vi "MainRIOEnrique.vi"() -> ()   [LabVIEW 2019]
uses:
  RIOData--cluster.ctl
  Acelerometer data--cluster.ctl
  <vilib>/PantherLAB/Firebase API/PantherLAB_lib_Filtering Parameters--cluster.ctl
  a087fea8-a487-4c1c-8a8b-15f205e78756.vi
  c90b4970-0cb1-4ed8-a3e8-abf7f56642d0.vi
  079ee137-338a-4224-8d27-3950f07d8dd5.vi
  <vilib>/JDP Science/JSONtext/JSON text to Variant.vi
  <vilib>/JDP Science/JSONtext/LVClass Serializer/JSONtext LVClass Serializer.lvclass
  <vilib>/PantherLAB/Firebase API/PantherLAB_lib_firebase.lvclass
  Shared.lvlib
  <vilib>/JDP Science/JSONtext/JSONtext.lvlib
panel:
  in  "Get All":bool
  in  "Get5":bool
  out "JSON String":string
  in  "Get Newest":bool
  in  "Delete":bool
  in  "Password":string="123456"
  in  "Email":string="enrique.noe@gmail.com"
  in  "Log In":bool
  in  "Sign In":bool
  out "Newest":T1
  out "Data out":T1[](array[typedef])
  out "My RIO Acelerometer":T2(graph)
  # "To add an authenticated user\nto your Real Time Database"
  # "If you are already authenticated\nand you want to start using\nyour Database"
  # "Warning:\nThis button will delete all the data\nunder Post EndPoint"
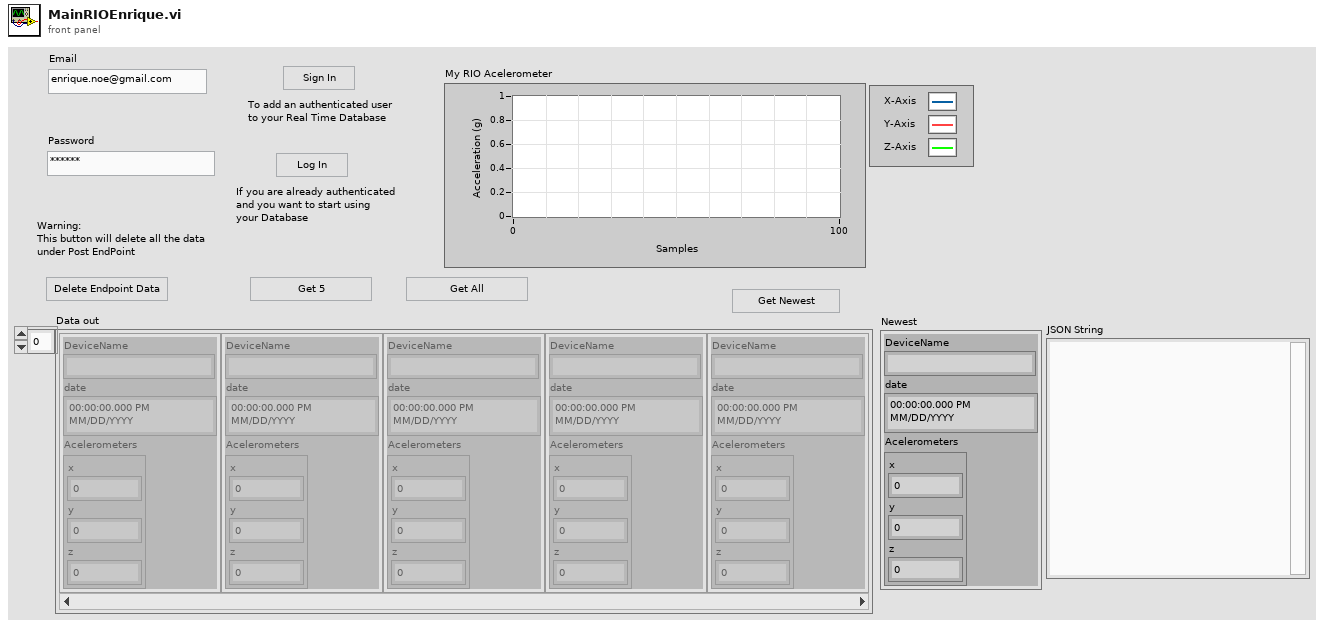
[diagram p1: front panel]
types:
  T1 = typedef "Shared.lvlib/RIOData--cluster.ctl" = cluster{"DeviceName":string, "date":timestamp, "Acelerometers":cluster{"x":dbl, "y":dbl, "z":dbl}}
  T2 = typedef "Shared.lvlib/Acelerometer data--cluster.ctl" = cluster{"X-Axis":dbl, "Y-Axis":dbl, "Z-Axis":dbl}
  T3 = cluster{"Read Access":enum8{"Allowed", "Required", "None"}, "Write Access":enum8{"Allowed", "Required", "None"}}
  T4 = typedef "PantherLAB_lib_firebase.lvclass/PantherLAB_lib_Filtering Parameters--cluster.ctl" = cluster{"Filtering Param":string, "Argument":string}
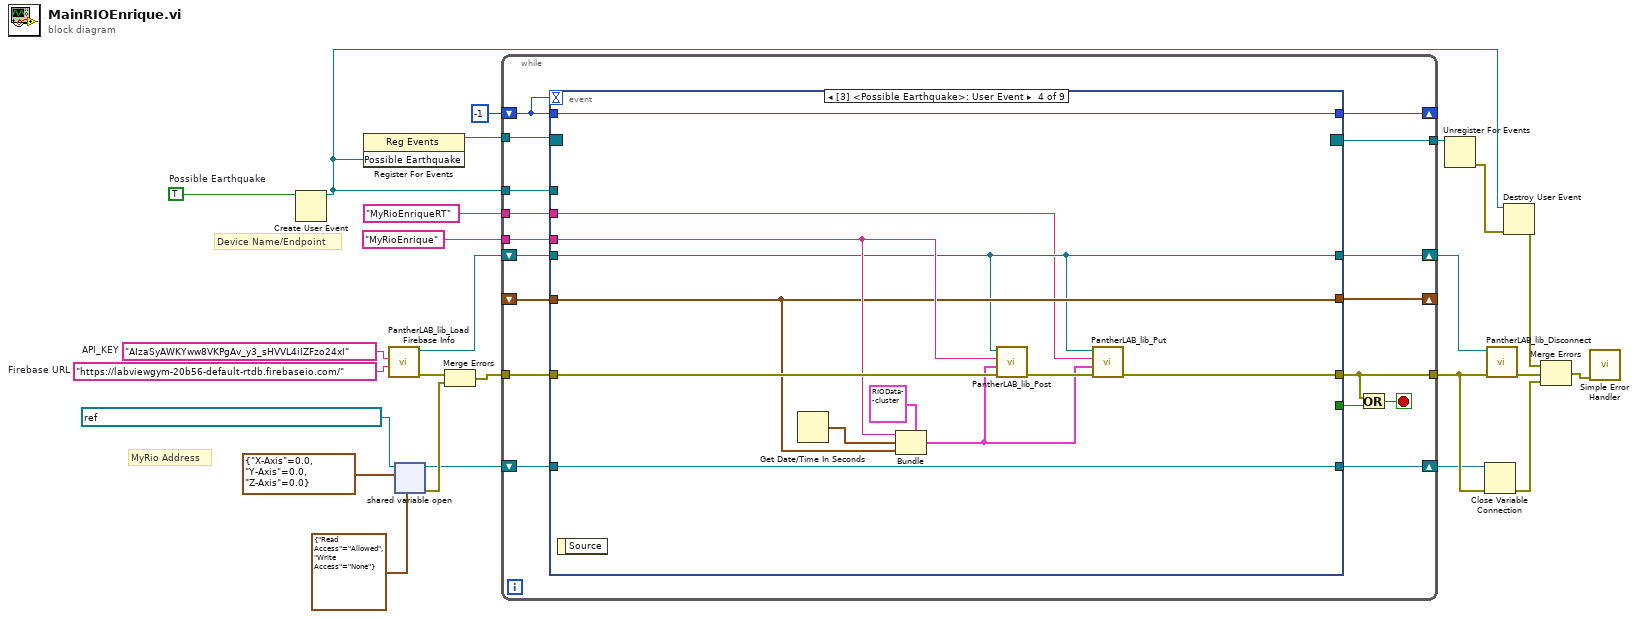
[diagram p0: block diagram]
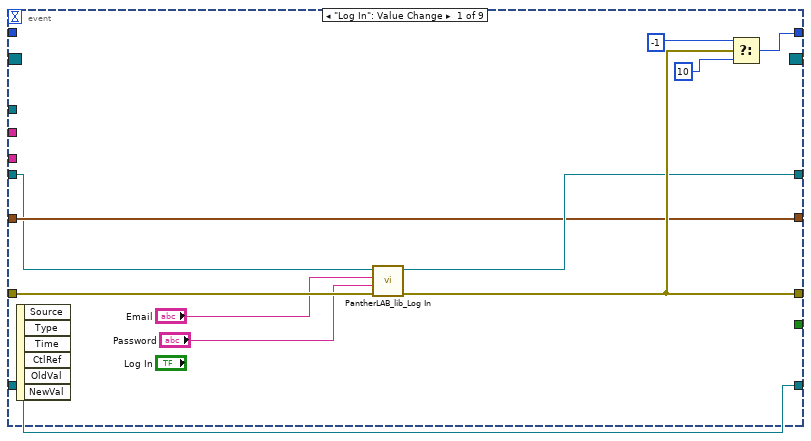
[diagram p2: hidden frame]
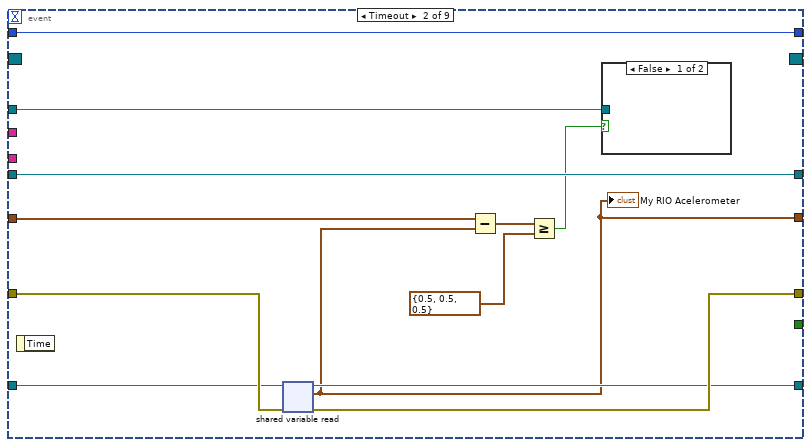
[diagram p3: hidden frame]
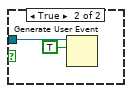
[diagram p4: hidden frame]
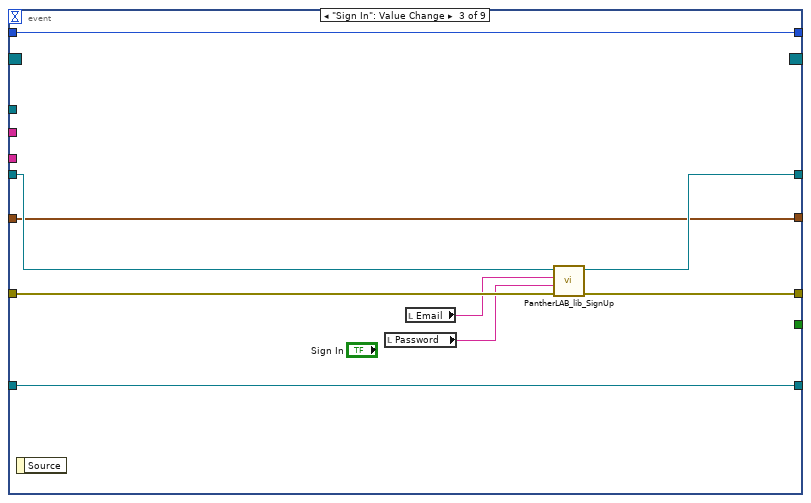
[diagram p5: hidden frame]
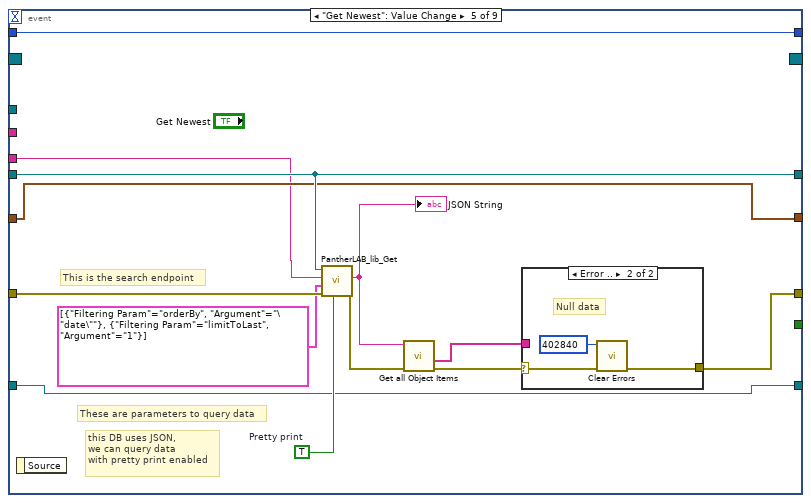
[diagram p6: hidden frame]
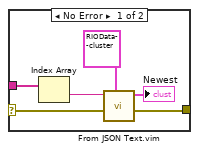
[diagram p7: hidden frame]
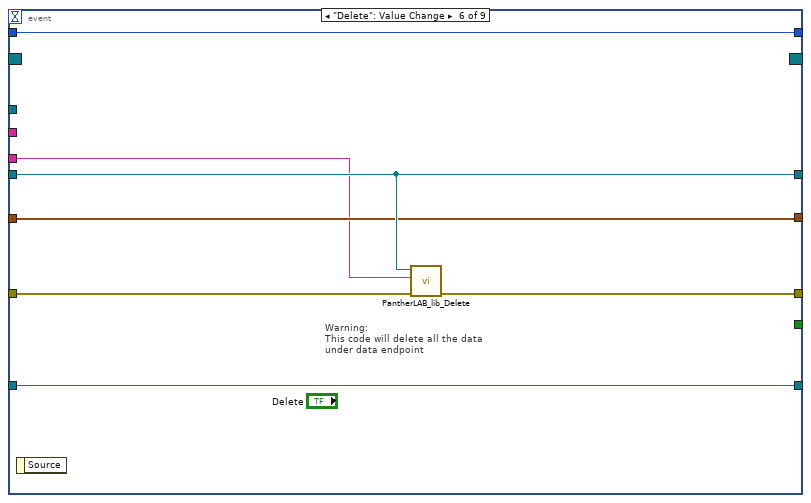
[diagram p8: hidden frame]
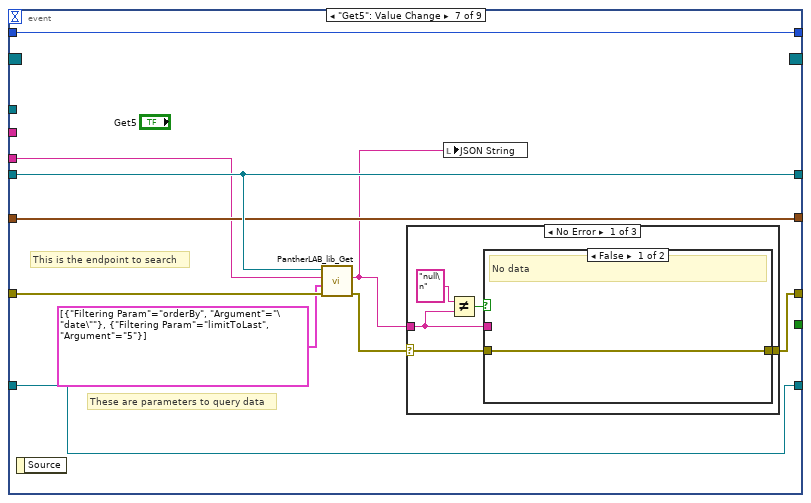
[diagram p9: hidden frame]
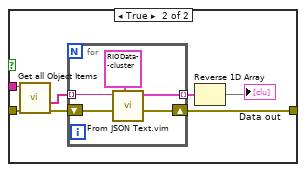
[diagram p10: hidden frame]
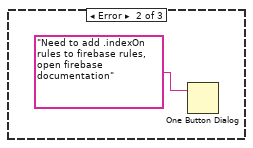
[diagram p11: hidden frame]
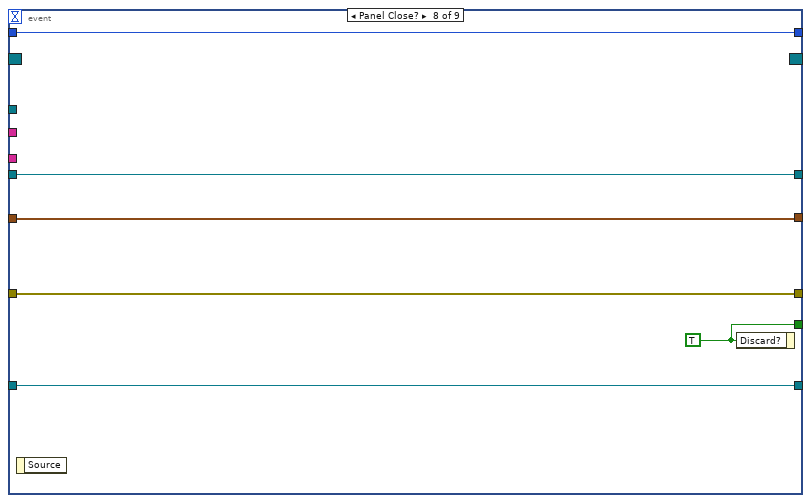
[diagram p13: hidden frame]
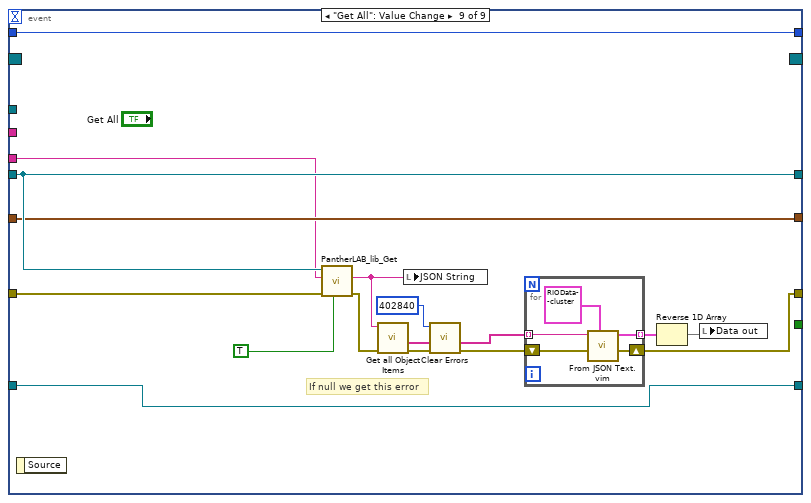
[diagram p14: hidden frame]
diagram:
  w6 = TRUE  # Possible Earthquake
  w11 = "AIzaSyAWKYww8VKPgAv_y3_sHVVL4iIZFzo24xI"  # API_KEY
  w10 = "https://labviewgym-20b56-default-rtdb.firebaseio.com/"  # Firebase URL
  # "MyRio Address"
  # "Device Name/Endpoint"
  n1 = Create User Event(user event datatype=w6) -> (user event=w4:refnum<user-event>)  [unwired: 1 in, 1 out]
  n2 = register-events(w4) -> (reference out=w7:refnum<event-registration>)  [unwired: 2 in, 1 out]
  n3 = call <vilib>:"PantherLAB_lib_Load Firebase Info.vi"("Firebase URL"=w10, "API_KEY"=w11) -> ("error out"=w24:errorcluster, "firebase out"=w12:refnum<class "PantherLAB_lib_firebase.lvclass">)  [unwired: 8 in]
  n4 = shared-variable-open(refnum<k21> "ni.var.psp://192.168.0.227/MyRioLib/AcelerationRIO" ("shared variable refnum in"), T2 {"X-Axis"=0.0, "Y-Axis"=0.0, "Z-Axis"=0.0} ("Acceleration"), T3 {"Read Access"=enum."Allowed", "Write Access"=enum."None"} ("access")) -> (w9:refnum<k21>, w22:errorcluster)  [unwired: 1 in]
  n5 = Merge Errors(w24, w22) -> (w23:errorcluster)
  n6 = while {
    tunnel: w23 -> [w42]
    tunnel: [w41] -> w21
    shift-right: [w37] -> w13
    shift-left: w12 -> [w38]
    shift-right: [w35] -> w8
    shift-left: w9 -> [w36]
    tunnel: w7 -> [w34]
    tunnel: w4 -> [w33]
    shift-right: [w32] -> _
    shift-left: _ -> [w31]
    tunnel: [w30] -> w5
    tunnel: "MyRioEnrique" -> [w29]
    shift-right: [w28] -> _
    shift-left: -1 -> [w27]
    tunnel: "MyRioEnriqueRT" -> [w26]
    stop <- w39 stop-if-true
    n7 = event shown="[3] <Possible Earthquake>: User Event" {
      selector: w34 -> [_ _ _ _ _ _ _ _ _]
      dyn-events: [_ _ _ _ _ _ _ _ _] -> w30
      timeout: w27 -> [_ _ _ _ _ _ _ _ _]
      tunnel: w42 -> [w53 w65 w76 w88 w101 w117 w127 w153 w169]
      tunnel: [w52 w64 w75 w86 w99 w116 w125 w153 w166] -> w41
      tunnel: [_ _ _ _ _ _ _ w151 _] -> w40
      tunnel: w38 -> [w46 w63 w72 w79 w94 w115 w123 w152 w159]
      tunnel: [w49 w63 w71 w79 w94 w115 w123 w152 w159] -> w37
      tunnel: w36 -> [w48 w62 w70 w85 w93 w114 w122 w150 w158]
      tunnel: [w48 w61 w70 w85 w93 w114 w122 w150 w158] -> w35
      tunnel: w33 -> [_ w58 _ _ _ _ _ _ _]
      tunnel: [w47 w56 w69 w81 w92 w113 w121 w149 w157] -> w32
      tunnel: w31 -> [w47 w57 w69 w81 w92 w113 w121 w149 w157]
      tunnel: w29 -> [_ _ _ w84 w91 w112 w120 _ w156]
      tunnel: [w43 w54 w68 w80 w89 w111 w118 w148 w154] -> w28
      tunnel: w27 -> [_ w54 w68 w80 w89 w111 w118 w148 w154]
      tunnel: w26 -> [_ _ _ w77 _ _ _ _ _]
      event "Log In": Value Change {
        n8 = event-data() -> ()  [unwired: 1 in, 6 out]
        n9 = call-dynamic "PantherLAB_lib_Log In.vi"("error in"=w53, "password"="Password", "email"="Email", "firebase in"=w46) -> ("error out"=w52:errorcluster, "firebase out"=w49:refnum<class "PantherLAB_lib_firebase.lvclass">)  [unwired: 6 in]
        n10 = Select(t=-1, s=w52, f=10) -> (s? t:f=w43:i32)
      }
      event Timeout {
        n11 = event-data() -> ()  [unwired: 1 in, 1 out]
        n12 = shared-variable-read(w62, w65) -> (w61:refnum<k21>, w64:errorcluster, w56:T2)  [unwired: 1 out]
        "My RIO Acelerometer" <- w56
        n13 = Subtract(x=w57, y=w56) -> (x-y=w60:T2)
        n14 = Greater Or Equal?(x=w60, y=T2 {"X-Axis"=0.5, "Y-Axis"=0.5, "Z-Axis"=0.5} ("x")) -> (x >= y?=w55:bool)
        n15 = case shown="False" w55 {
          tunnel: w58 -> [_ w67]
          frame False {
          }
          frame True {
            n16 = Generate User Event(user event=w67, event data cluster=TRUE ("event data")) -> ()  [unwired: 2 in, 2 out]
          }
        }
      }
      event "Sign In": Value Change {
        n17 = event-data() -> ()  [unwired: 1 in, 1 out]
        n18 = local read "Password"() -> (w74:string)
        n19 = local read "Email"() -> (w73:string)
        n20 = call-dynamic "PantherLAB_lib_SignUp.vi"("error in"=w76, "password"=w74, "email"=w73, "firebase in"=w72) -> ("error out"=w75:errorcluster, "firebase out"=w71:refnum<class "PantherLAB_lib_firebase.lvclass">)  [unwired: 6 in]
      }
      event User Event {
        n21 = event-data() -> ()  [unwired: 1 in, 1 out]
        n22 = Get Date/Time In Seconds() -> (seconds since 1Jan1904=w83:timestamp)
        n23 = Bundle(cluster=T1 {"DeviceName"="", "date"=timestamp(0 s since 1904-01-01), "Acelerometers"={"x"=0.0, "y"=0.0, "z"=0.0}} ("output cluster"), "DeviceName"=w84, "date"=w83, "Acelerometers"=w81) -> (w78:T1)
        n24 = call-dynamic "PantherLAB_lib_Post.vi"("error in"=w88, "Anything"=w78, "endPoint"=w84, "firebase in"=w79) -> ("error out"=w87:errorcluster)  [unwired: 6 in, 1 out]
        n25 = call-dynamic "PantherLAB_lib_Put.vi"("error in"=w87, "Anything"=w78, "endPoint"=w77, "firebase in"=w79) -> ("error out"=w86:errorcluster)  [unwired: 6 in, 1 out]
      }
      event "Get Newest": Value Change {
        w95 = TRUE  # Pretty print
        # "this DB uses JSON,\nwe can query data\nwith pretty print enabled"
        # "These are parameters to query data"
        # "This is the search endpoint"
        n26 = event-data() -> ()  [unwired: 1 in, 1 out]
        n27 = call-dynamic "PantherLAB_lib_Get.vi"("Pretty print"=w95, "error in"=w101, "Filtering Params"=T4[] [{"Filtering Param"="orderBy", "Argument"="\"date\""}, {"Filtering Param"="limitToLast", "Argument"="1"}], "endPoint"=w91, "firebase in"=w94) -> ("error out"=w100:errorcluster, "Json String"=w96:string)  [unwired: 5 in]
        "JSON String" <- w96
        n28 = call <vilib>:"Get all Object Items.vi"("error in (no error)"=w100, "JSON"=w96) -> ("error out"=w98:errorcluster, "<JSON>"=w90:string[])  [unwired: 6 in, 2 out]
        n29 = case shown="Error .." w98 {
          selector: w98 -> [w107 w110]
          tunnel: [w106 w109] -> w99
          tunnel: w90 -> [w105 _]
          frame No Error {
            n30 = Index Array(array=w105) -> (element=w104:string)  [unwired: 1 in]
            n31 = call "From JSON Text.vim"("Data Type and Default Value"=T1 {"DeviceName"="", "date"=timestamp(0 s since 1904-01-01), "Acelerometers"={"x"=0.0, "y"=0.0, "z"=0.0}} ("Array"), "error in (no error)"=w107, "JSON"=w104) -> ("error out"=w106:errorcluster, "Data out"=→"Newest":T1)  [unwired: 7 in]
          }
          frame Error {
            # "Null data"
            n32 = call <vilib>:"Clear Errors.vi"("error in (no error)"=w110, "specific error code to clear (0: all)"=402840) -> ("error out"=w109:errorcluster)  [unwired: 4 in, 1 out]
          }
        }
      }
      event "Delete": Value Change {
        # "Warning:\nThis code will delete all the data\nunder data endpoint"
        n33 = event-data() -> ()  [unwired: 1 in, 1 out]
        n34 = call-dynamic "PantherLAB_lib_Delete.vi"("error in"=w117, "endPoint"=w112, "firebase in"=w115) -> ("error out"=w116:errorcluster)  [unwired: 7 in, 1 out]
      }
      event "Get5": Value Change {
        # "This is the endpoint to search"
        # "These are parameters to query data"
        n35 = event-data() -> ()  [unwired: 1 in, 1 out]
        n36 = call-dynamic "PantherLAB_lib_Get.vi"("error in"=w127, "Filtering Params"=T4[] [{"Filtering Param"="orderBy", "Argument"="\"date\""}, {"Filtering Param"="limitToLast", "Argument"="5"}], "endPoint"=w120, "firebase in"=w123) -> ("error out"=w126:errorcluster, "Json String"=w119:string)  [unwired: 6 in]
        n37 = case shown="No Error" w126 {
          selector: w126 -> [w132 _ w147]
          tunnel: [w131 _ w147] -> w125
          tunnel: w119 -> [w128 _ _]
          frame No Error {
            n38 = Not Equal?(x="null\n" ("Display"), y=w128) -> (x != y?=w129:bool)
            n39 = case shown="False" w129 {
              tunnel: w132 -> [w133 w139]
              tunnel: [w133 w138] -> w131
              tunnel: w128 -> [_ w135]
              frame False {
                # "No data"
              }
              frame True {
                n40 = call <vilib>:"Get all Object Items.vi"("error in (no error)"=w139, "JSON"=w135) -> ("error out"=w140:errorcluster, "<JSON>"=w137:string[])  [unwired: 6 in, 2 out]
                n41 = for {
                  tunnel: w137 -> [w143] mode=indexing
                  shift-right: [w144] -> w138
                  shift-left: w140 -> [w145]
                  tunnel: [w142] -> w136 mode=indexing
                  n42 = call "From JSON Text.vim"("Data Type and Default Value"=T1 {"DeviceName"="", "date"=timestamp(0 s since 1904-01-01), "Acelerometers"={"x"=0.0, "y"=0.0, "z"=0.0}} ("RioData"), "error in (no error)"=w145, "JSON"=w143) -> ("error out"=w144:errorcluster, "Data out"=w142:T1)  [unwired: 7 in]
                }
                n43 = Reverse 1D Array(array=w136) -> (reversed array=→"Data out":T1[])
              }
            }
          }
          frame Error {
            n44 = One Button Dialog(message="Need to add .indexOn rules to firebase rules, open firebase documentation") -> ()  [unwired: 1 in, 1 out]
          }
          frame Default {
          }
        }
        n45 = local write "JSON String"(w119) -> ()
      }
      event Panel Close? {
        w151 = TRUE ("Discard?")
        n46 = event-data() -> ()  [unwired: 1 in, 1 out]
        n47 = event-data("Discard?"=w151) -> ()  [unwired: 1 in, 1 out]
      }
      event "Get All": Value Change {
        # "If null we get this error"
        n48 = event-data() -> ()  [unwired: 1 in, 1 out]
        n49 = call-dynamic "PantherLAB_lib_Get.vi"("Pretty print"=TRUE, "error in"=w169, "endPoint"=w156, "firebase in"=w159) -> ("error out"=w167:errorcluster, "Json String"=w162:string)  [unwired: 6 in]
        n50 = call <vilib>:"Get all Object Items.vi"("error in (no error)"=w167, "JSON"=w162) -> ("error out"=w168:errorcluster, "<JSON>"=w164:string[])  [unwired: 6 in, 2 out]
        n51 = local write "JSON String"(w162) -> ()
        n52 = call <vilib>:"Clear Errors.vi"("error in (no error)"=w168, "specific error code to clear (0: all)"=402840) -> ("error out"=w165:errorcluster)  [unwired: 4 in, 1 out]
        n53 = for {
          tunnel: w164 -> [w172] mode=indexing
          shift-right: [w173] -> w166
          shift-left: w165 -> [w174]
          tunnel: [w171] -> w163 mode=indexing
          n54 = call "From JSON Text.vim"("Data Type and Default Value"=T1 {"DeviceName"="", "date"=timestamp(0 s since 1904-01-01), "Acelerometers"={"x"=0.0, "y"=0.0, "z"=0.0}} ("RioData"), "error in (no error)"=w174, "JSON"=w172) -> ("error out"=w173:errorcluster, "Data out"=w171:T1)  [unwired: 7 in]
        }
        n55 = Reverse 1D Array(array=w163) -> (reversed array=w155:T1[])
        n56 = local write "Data out"(w155) -> ()
      }
    }
    n57 = Or(x=w41, y=w40) -> (x .or. y?=w39:bool)
  }
  n58 = Unregister For Events(event registration refnum=w5) -> (error out=w17:errorcluster)  [unwired: 1 in]
  n59 = Close Variable Connection(8:w21, 11:w8) -> (0:w19:errorcluster)
  n60 = call-dynamic "PantherLAB_lib_Disconnect.vi"("error in"=w21, "firebase in"=w13) -> ("error out"=w25:errorcluster)  [unwired: 9 in]
  n61 = Destroy User Event(user event=w4, error in=w17) -> (error out=w18:errorcluster)
  n62 = Merge Errors(w18, w25, w19) -> (w20:errorcluster)
  n63 = call <vilib>:"Simple Error Handler.vi"("error in (no error)"=w20) -> ()  [unwired: 4 in, 5 out]
